vi "Compute boxplot data.vi"(6 "Box Width":dbl=10.0 format="%.2f", 9 "Plot #":u32, 10 "Raw Data":dbl[](array[numeric]) format="%.2f") -> (0 "min":dbl, 1 "max":dbl, 2 "XY Graph":cluster{dbl[], dbl[]}[](graph))   [LabVIEW 2022 SP3, in "Box Plots.lvlib"]
doc: "Computes the xy graph data points necessary to draw a box plot on a XY graph."
uses:
  Box Plots.lvlib
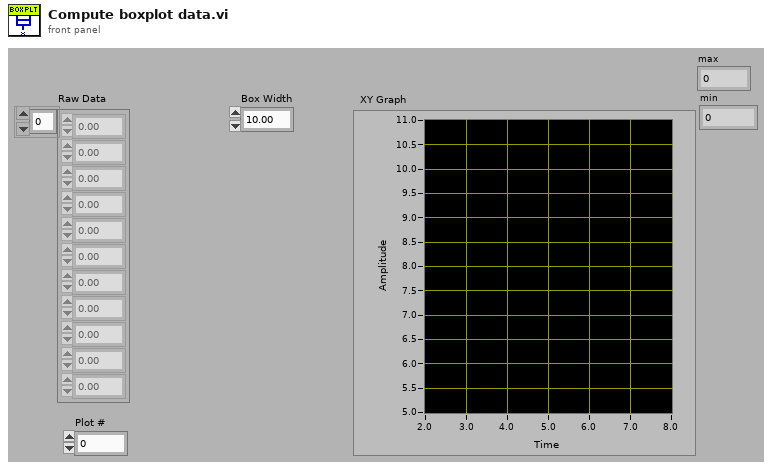
[diagram p1: front panel]
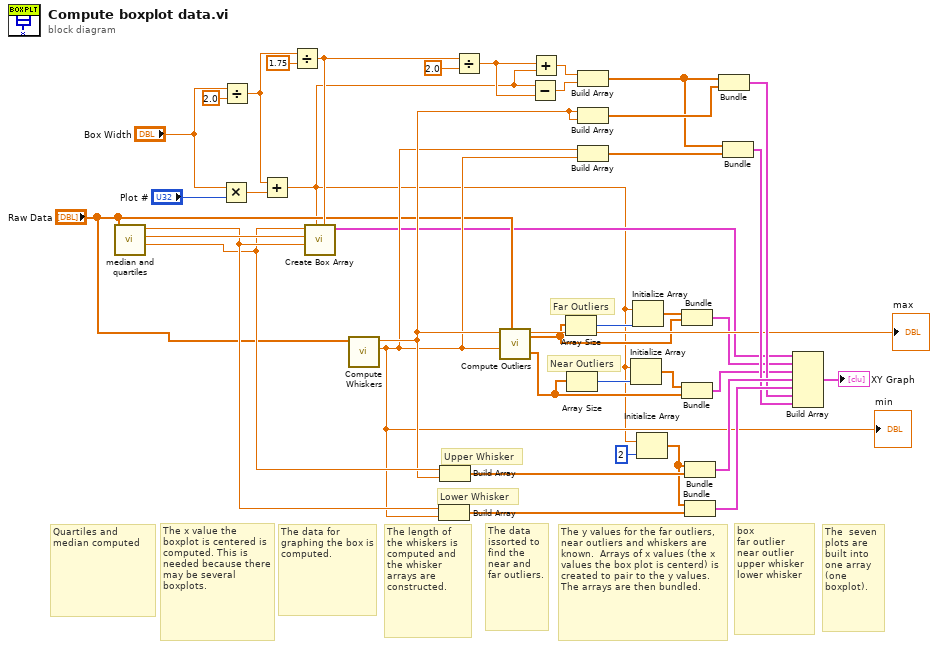
[diagram p0: block diagram]
diagram:
  # "Near Outliers"
  # "Far Outliers"
  # "box\nfar outlier\nnear outlier\nupper whisker\nlower whisker"
  # "The data issorted to find the near and far outliers."
  # "The length of the whiskers is computed and the whisker arrays are constructed."
  # "The data for graphing the box is computed."
  # "The x value the boxplot is centered is computed. This is needed because there may be several boxplots."
  # "Quartiles and median computed"
  # "The  seven plots are built into one array (one boxplot)."
  # "The y values for the far outliers, near outliers and whiskers are known.  Arrays of x values (the x values the box plot is centerd) is created to pair to the y values.  The arrays are then bundled."
  # "Lower Whisker"
  # "Upper Whisker"
  n1 = call "median and quartiles.vi"("data"="Raw Data") -> ("Q3"=w15:dbl, "median"=w32:dbl, "Q1"=w16:dbl)  [unwired: 6 out]
  n2 = Multiply(x="Box Width", y="Plot #") -> (x*y=w31:dbl)
  n3 = Divide(x="Box Width", y=2.0 ("x")) -> (x/y=w18:dbl)
  n4 = Add(x=w18, y=w31) -> (x+y=w1:dbl)
  n5 = Divide(x=w18, y=1.75 ("x")) -> (x/y=w17:dbl)
  n6 = call "Create Box Array.vi"("Box Width"=w17, "X position"=w1, "Lower Quartile (LQ)"=w16, "Median"=w32, "Upper Quartile (UQ)"=w15) -> ("XY Graph"=w6:cluster{dbl[], dbl[]})  [unwired: 6 in]
  n7 = call "Compute Whiskers.vi"("ORIGINAL ARRAY"="Raw Data") -> ("min"=w12:dbl, "max"=w13:dbl)  [unwired: 3 in, 2 out]
  "max" <- w13
  "min" <- w12
  n8 = Build Array(w16, w12) -> (w37:dbl[])
  n9 = Build Array(w15, w13) -> (w38:dbl[])
  n10 = Divide(x=w17, y=2.0) -> (x/y=w25:dbl)
  n11 = call "Compute Outliers.vi"("U1"=w13, "L1"=w12, "Raw Data"="Raw Data") -> ("Far Outliers"=w5:dbl[], "Near Outliers"=w4:dbl[])  [unwired: 2 in]
  n12 = Subtract(x=w1, y=w25) -> (x-y=w26:dbl)
  n13 = Add(x=w25, y=w1) -> (x+y=w27:dbl)
  n14 = Array Size(array=w5) -> (size(s)=w10:i32)
  n15 = Array Size(array=w4) -> (size(s)=w9:i32)
  n16 = Build Array(w27, w26) -> (w23:dbl[])
  n17 = Build Array(w13, w13) -> (w24:dbl[])
  n18 = Build Array(w12, w12) -> (w22:dbl[])
  n19 = Initialize Array(w1, w9) -> (w7:dbl[])
  n20 = Initialize Array(w1, w10) -> (w8:dbl[])
  n21 = Initialize Array(w1, 2 ("dimension size")) -> (w36:dbl[])
  n22 = Bundle(w8, "Far Outliers"=w5) -> (w3:cluster{dbl[], "Far Outliers":dbl[]})  [unwired: 1 out]
  n23 = Bundle(w7, "Near Outliers"=w4) -> (w2:cluster{dbl[], "Near Outliers":dbl[]})  [unwired: 1 out]
  n24 = Bundle(w36, w38) -> (w35:cluster{dbl[], dbl[]})  [unwired: 1 out]
  n25 = Bundle(w36, w37) -> (w34:cluster{dbl[], dbl[]})  [unwired: 1 out]
  n26 = Bundle(w23, w24) -> (w30:cluster{dbl[], dbl[]})  [unwired: 1 out]
  n27 = Bundle(w23, w22) -> (w14:cluster{dbl[], dbl[]})  [unwired: 1 out]
  n28 = Build Array(w6, w3, w2, w35, w34, w30, w14) -> (→"XY Graph":cluster{dbl[], "Near Outliers":dbl[]}[])
